vi "read root dir.vi"(8 "error in (no error)":errorcluster, 11 "TCP in":refnum<k5>) -> (0 "error out":errorcluster, 2 "root elements":T1[](array[typedef]), 3 "TCP out":refnum<k5>)   [LabVIEW 2020]
uses:
  ctl/9-id,name,path.ctl
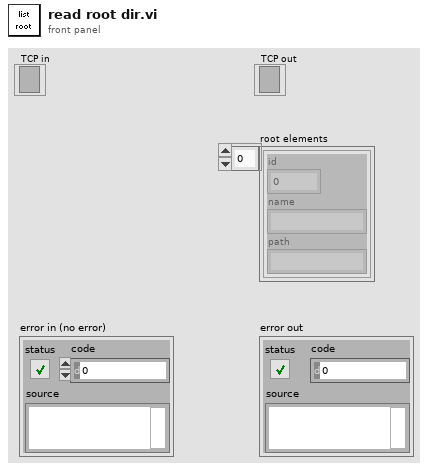
[diagram p1: front panel]
types:
  T1 = typedef "9-id,name,path.ctl" = cluster{"id":u8, "name":string, "path":string}
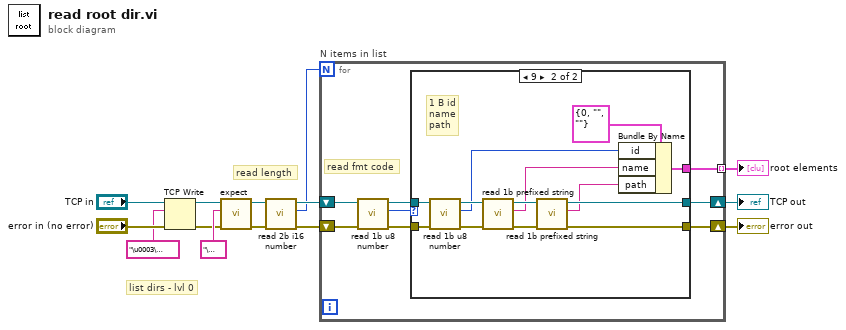
[diagram p0: block diagram]
diagram:
  # "read length"
  # "list dirs - lvl 0"
  n1 = TCP Write(connection ID="TCP in", data in="\u0003\u0000\u0000", error in (no error)="error in (no error)") -> (connection ID out=w8:refnum<k5>, error out=w5:errorcluster)  [unwired: 1 in, 1 out]
  n2 = call "expect.vi"("error in (no error)"=w5, "data expected"="\u0001" ("data in"), "TCP Network Connection in"=w8) -> ("error out"=w7:errorcluster, "TCP Network Connection out"=w2:refnum<k5>)  [unwired: 6 in, 1 out]
  n3 = call "read 2b i16 number.vi"("error in (no error)"=w7, "TCP Network Connection in"=w2) -> ("error out"=w10:errorcluster, "number"=w1:i16, "TCP Network Connection out"=w11:refnum<k5>)  [unwired: 7 in]
  n4 = for "N items in list" {
    N: w1 -> [_]
    shift-right: [w17] -> w13
    shift-left: w11 -> [w22]
    shift-right: [w19] -> w12
    shift-left: w10 -> [w21]
    tunnel: [w15] -> w14 mode=indexing
    # "read fmt code"
    n5 = call "read 1b u8 number.vi"("error in (no error)"=w21, "TCP Network Connection in"=w22) -> ("error out"=w20:errorcluster, "number"=w16:u8, "TCP Network Connection out"=w18:refnum<k5>)  [unwired: 7 in]
    n6 = case shown="9" w16 {
      tunnel: w20 -> [w23 w37]
      tunnel: [w23 w30] -> w19
      tunnel: w18 -> [w24 w32]
      tunnel: [w24 w28] -> w17
      tunnel: [_ w34] -> w15
      frame Default {
      }
      frame 9 {
        # "1 B id\nname\npath"
        n7 = call "read 1b u8 number.vi"("error in (no error)"=w37, "TCP Network Connection in"=w32) -> ("error out"=w33:errorcluster, "number"=w27:u8, "TCP Network Connection out"=w31:refnum<k5>)  [unwired: 7 in]
        n8 = call "read 1b prefixed string.vi"("error in (no error)"=w33, "TCP Network Connection in"=w31) -> ("error out"=w36:errorcluster, "data out"=w26:string, "TCP Network Connection out"=w29:refnum<k5>)  [unwired: 7 in]
        n9 = call "read 1b prefixed string.vi"("error in (no error)"=w36, "TCP Network Connection in"=w29) -> ("error out"=w30:errorcluster, "data out"=w25:string, "TCP Network Connection out"=w28:refnum<k5>)  [unwired: 7 in]
        n10 = Bundle By Name(cluster=T1 {"id"=0, "name"="", "path"=""} ("9 - id, len, data"), "id"=w27, "name"=w26, "path"=w25) -> (w34:T1)
      }
    }
  }
  "root elements" <- w14
  "TCP out" <- w13
  "error out" <- w12
